vi "shutter_switch.vi"(9 "COM":bool, 10 "VISA name":refnum<visa-resource-name>, 11 "eSwitchType 0 or 1":u8) -> (3 "return":i32)   [LabVIEW 2016]
panel:
  in  "tVdCmdHeader":T1
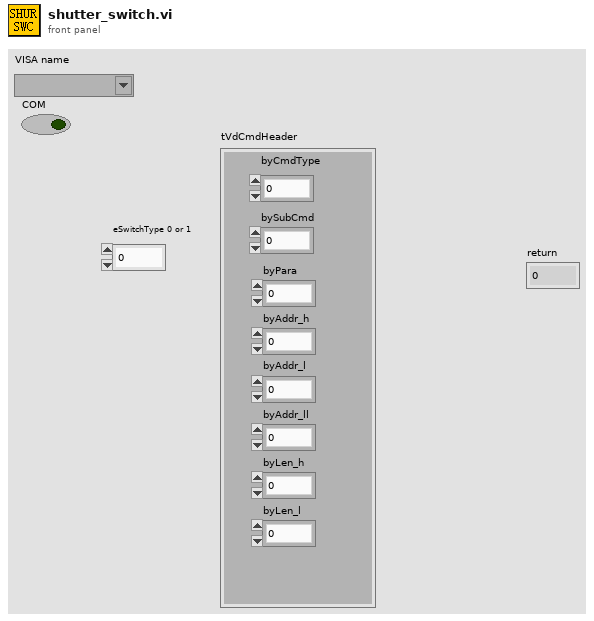
[diagram p1: front panel]
types:
  T1 = cluster{"byCmdType":u8, "bySubCmd":u8, "byPara":u8, "byAddr_h":u8, "byAddr_l":u8, "byAddr_ll":u8, "byLen_h ":u8, "byLen_l":u8}
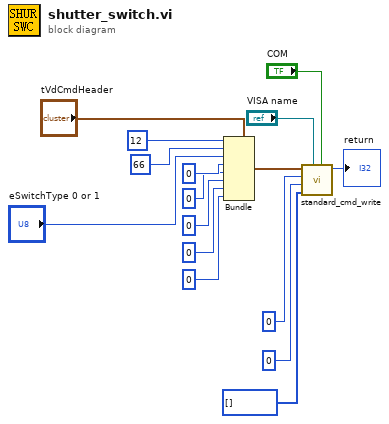
[diagram p0: block diagram]
diagram:
  n1 = Bundle(cluster="tVdCmdHeader", "byCmdType"=u8 12, "bySubCmd"=u8 66, "byPara"="eSwitchType 0 or 1", "byAddr_h"=u8 0, "byAddr_l"=u8 0, "byAddr_ll"=u8 0, "byLen_h"=u8 0, "byLen_l"=u8 0) -> (w13:T1)
  n2 = call "standard_cmd_write.vi"("COM"="COM", "VISA name"="VISA name", "data"=u8[] [], "dwLen"=u32 0, "dwAddr"=u32 0, "cmd_std_header_t"=w13) -> ("return"=→"return":i32)  [unwired: 5 in]
